vi "AO CorrLoop_PD_2D_v1.vi"() -> ()   [LabVIEW 2018]
uses:
  Casao LabVIEW SDK 1.0.5/Casao/Casao/Casao.ctl
  <vilib>/Analysis/1siggen.llb/Ramp Pattern by Samples.vi
  <vilib>/Utility/file.llb/Read From Spreadsheet File (DBL).vi
  <vilib>/Analysis/1siggen.llb/Ramp Pattern by Delta.vi
  <vilib>/Analysis/NI_AALBase.lvlib
panel:
  in  "Output Path 2":path=path "F:/Data_Min"
  in  "Trigger EMCCD":bool
  out "Tab Control":T1(tab)
  in  "Haso configuration file":path=path "C:/Program Files (x86)/Imagine Optic/Configuration Files/HASO3_first_7364.dat"
  in  "Offset command file":path=path "D:/SystemAlignment/system_aberration_20200627.dat"
  in  "Initial haso file":path=path "D:/SystemAlignment/system_aberration_residual_20200711.has"
  in  "EMCCD trigger port":tag="Dev1/port0/line0"
  out "Casao Index":T2
  out "# of Phase":i32
  in  "Error in":errorcluster
  in  "COMMAND matrix file":path=path "D:/SystemAlignment/CM_20200711_0p5x6.aomc"
  out "Error out":errorcluster
  in  "Diversity Zern Coeffs":enum16{"Manual ", "ZernFile"}(ring)=enum."ZernFile"
  in  "Zern coeffs initial":dbl[](array[numeric])=[0.3, 0.0]
  in  "Zern index initial":dbl[](array[numeric])=[4.0, 0.0]
  out "Zern coeffs (random)":dbl[](array[numeric])
  out "Zern index  (random from 4th)":dbl[](array[numeric])
  in  "aberration tolerance":dbl=0.1 format="%#_13g"
  in  "aberration threshold":dbl=0.25 format="%#_13g"
  in  "Initial Zern Coeffs":enum16{"Manual ", "Random"}(ring)
  in  "max random index":i64=9
  in  "Exp Repeat Num":i32=1
  in  "Coeffs 5":sgl[](array[numeric])=[-0.2, 0.5, 0.0, 0.0, 0.0, -0.2]
  in  "Index 5":i32[](array[numeric])=[3, 4, 5, 6, 7, 8]
  in  "Coeffs 4":sgl[](array[numeric])=[0.2, -0.5, 0.0, 0.0, 0.0, 0.0]
  in  "Index 4":i32[](array[numeric])=[3, 4, 5, 6, 7, 8]
  in  "Coeffs 3":sgl[](array[numeric])=[-0.2, -0.5, 0.0, 0.0, 0.0, 0.0]
  in  "Index 3":i32[](array[numeric])=[3, 4, 5, 6, 7, 8]
  in  "Coeffs 2":sgl[](array[numeric])=[0.2, 0.5, 0.0, 0.0, 0.0, 0.0]
  in  "Index 2":i32[](array[numeric])=[3, 4, 5, 6, 7, 8]
  in  "Zern coeffs file":path=path "D:/SystemAlignment/system_aberration_residual_20200711.txt"
  in  "Subfolder":string="Sample1"
  out "RMSE Value":dbl
  out "Time cost (s)":dbl
  in  "Folder Name":string="Test"
  in  "Main Path":path=path "D:/Data"
  in  "File Base Name":string="beads_test"
  in  "Images/phase":dbl=1.0
  in  "Exposure time (s)":string="0.02"
  in  "Num of Accumulations":string="1"
  in  "Diversity Phase Num":i32=2
  in  "ROI size":enum16{"full (1002*1002)", "512*512"}(ring)
  in  "take offset image?":bool=TRUE
  in  "Keep Reconstructed Defocus component?":bool caption="Apply Defocus"
  in  "PD Correction":bool=TRUE
  in  "Calculation Phase Num":u32=2
  in  "Number for average":u32=1
  in  "Zernike Index Limit":u32=21
  in  "Iteration Number":u32=10
  in  "Gamma Value":dbl=1e-06
  in  "Crop Size of image":u32=512
  in  "Background Value":u32=310
  in  "Show Input":bool
  in  "Show Recon":bool=TRUE
  in  "Use GPU":bool=TRUE
  # "AO correction loop based on phase diversity: 2D image case\nVersion 1: A combination of LabVIEW, MATLAB, and Andor software(by triggers)\n1) Replaced CASAO SDK function by new WaveTune SDK function;\n2) Reorgized UI and file/folder name;\n3) New PD recon MATLAB code (termination criterion)"
  # "How to use (date: 20200711)\n1) Run this VI;\n2) Run Andor script: AO CorrLoop_PD_2D_v1_Script\n3) Click \"Start Acquisition\" button."
  # "Manual input"
  # "Random input"
  # "Manual input sequence"
  # "File input"
  # "Path and File Name"
  # "Camera Preview"
  # "Andor EMCCD Settings"
  # "Module to add"
  # "Image Metrics"
  # "MATLAB Settings"
  # "Module to add"
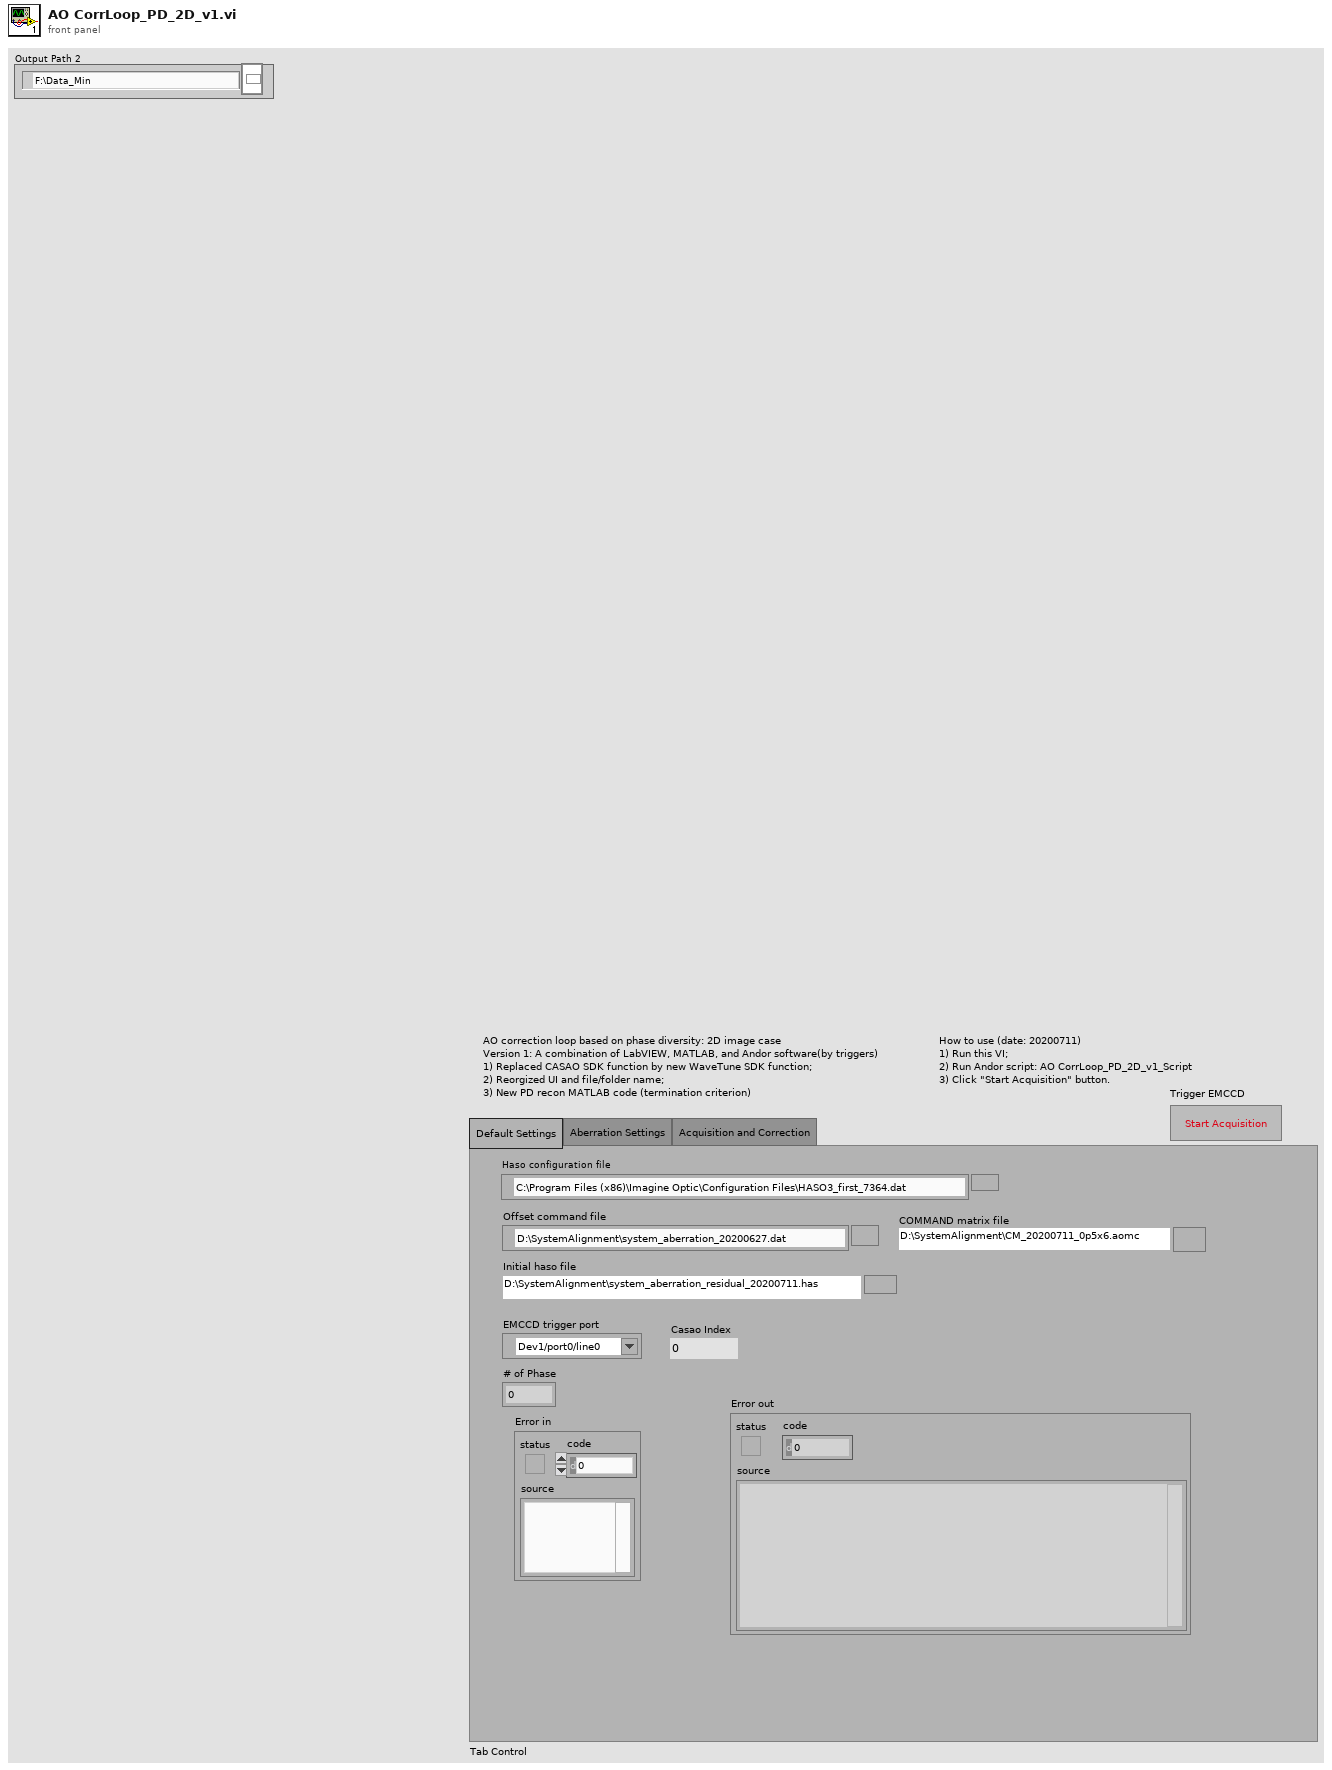
[diagram p1: front panel]
types:
  T1 = enum32{"Default Settings", "Aberration Settings", "Acquisition and Correction"}
  T2 = typedef "Casao.ctl" = i32
  T3 = typedef "PhaseModul.ctl" = i32
  T4 = typedef "NI_Matrix.lvlib/RealMatrix.ctl" = dbl[][]
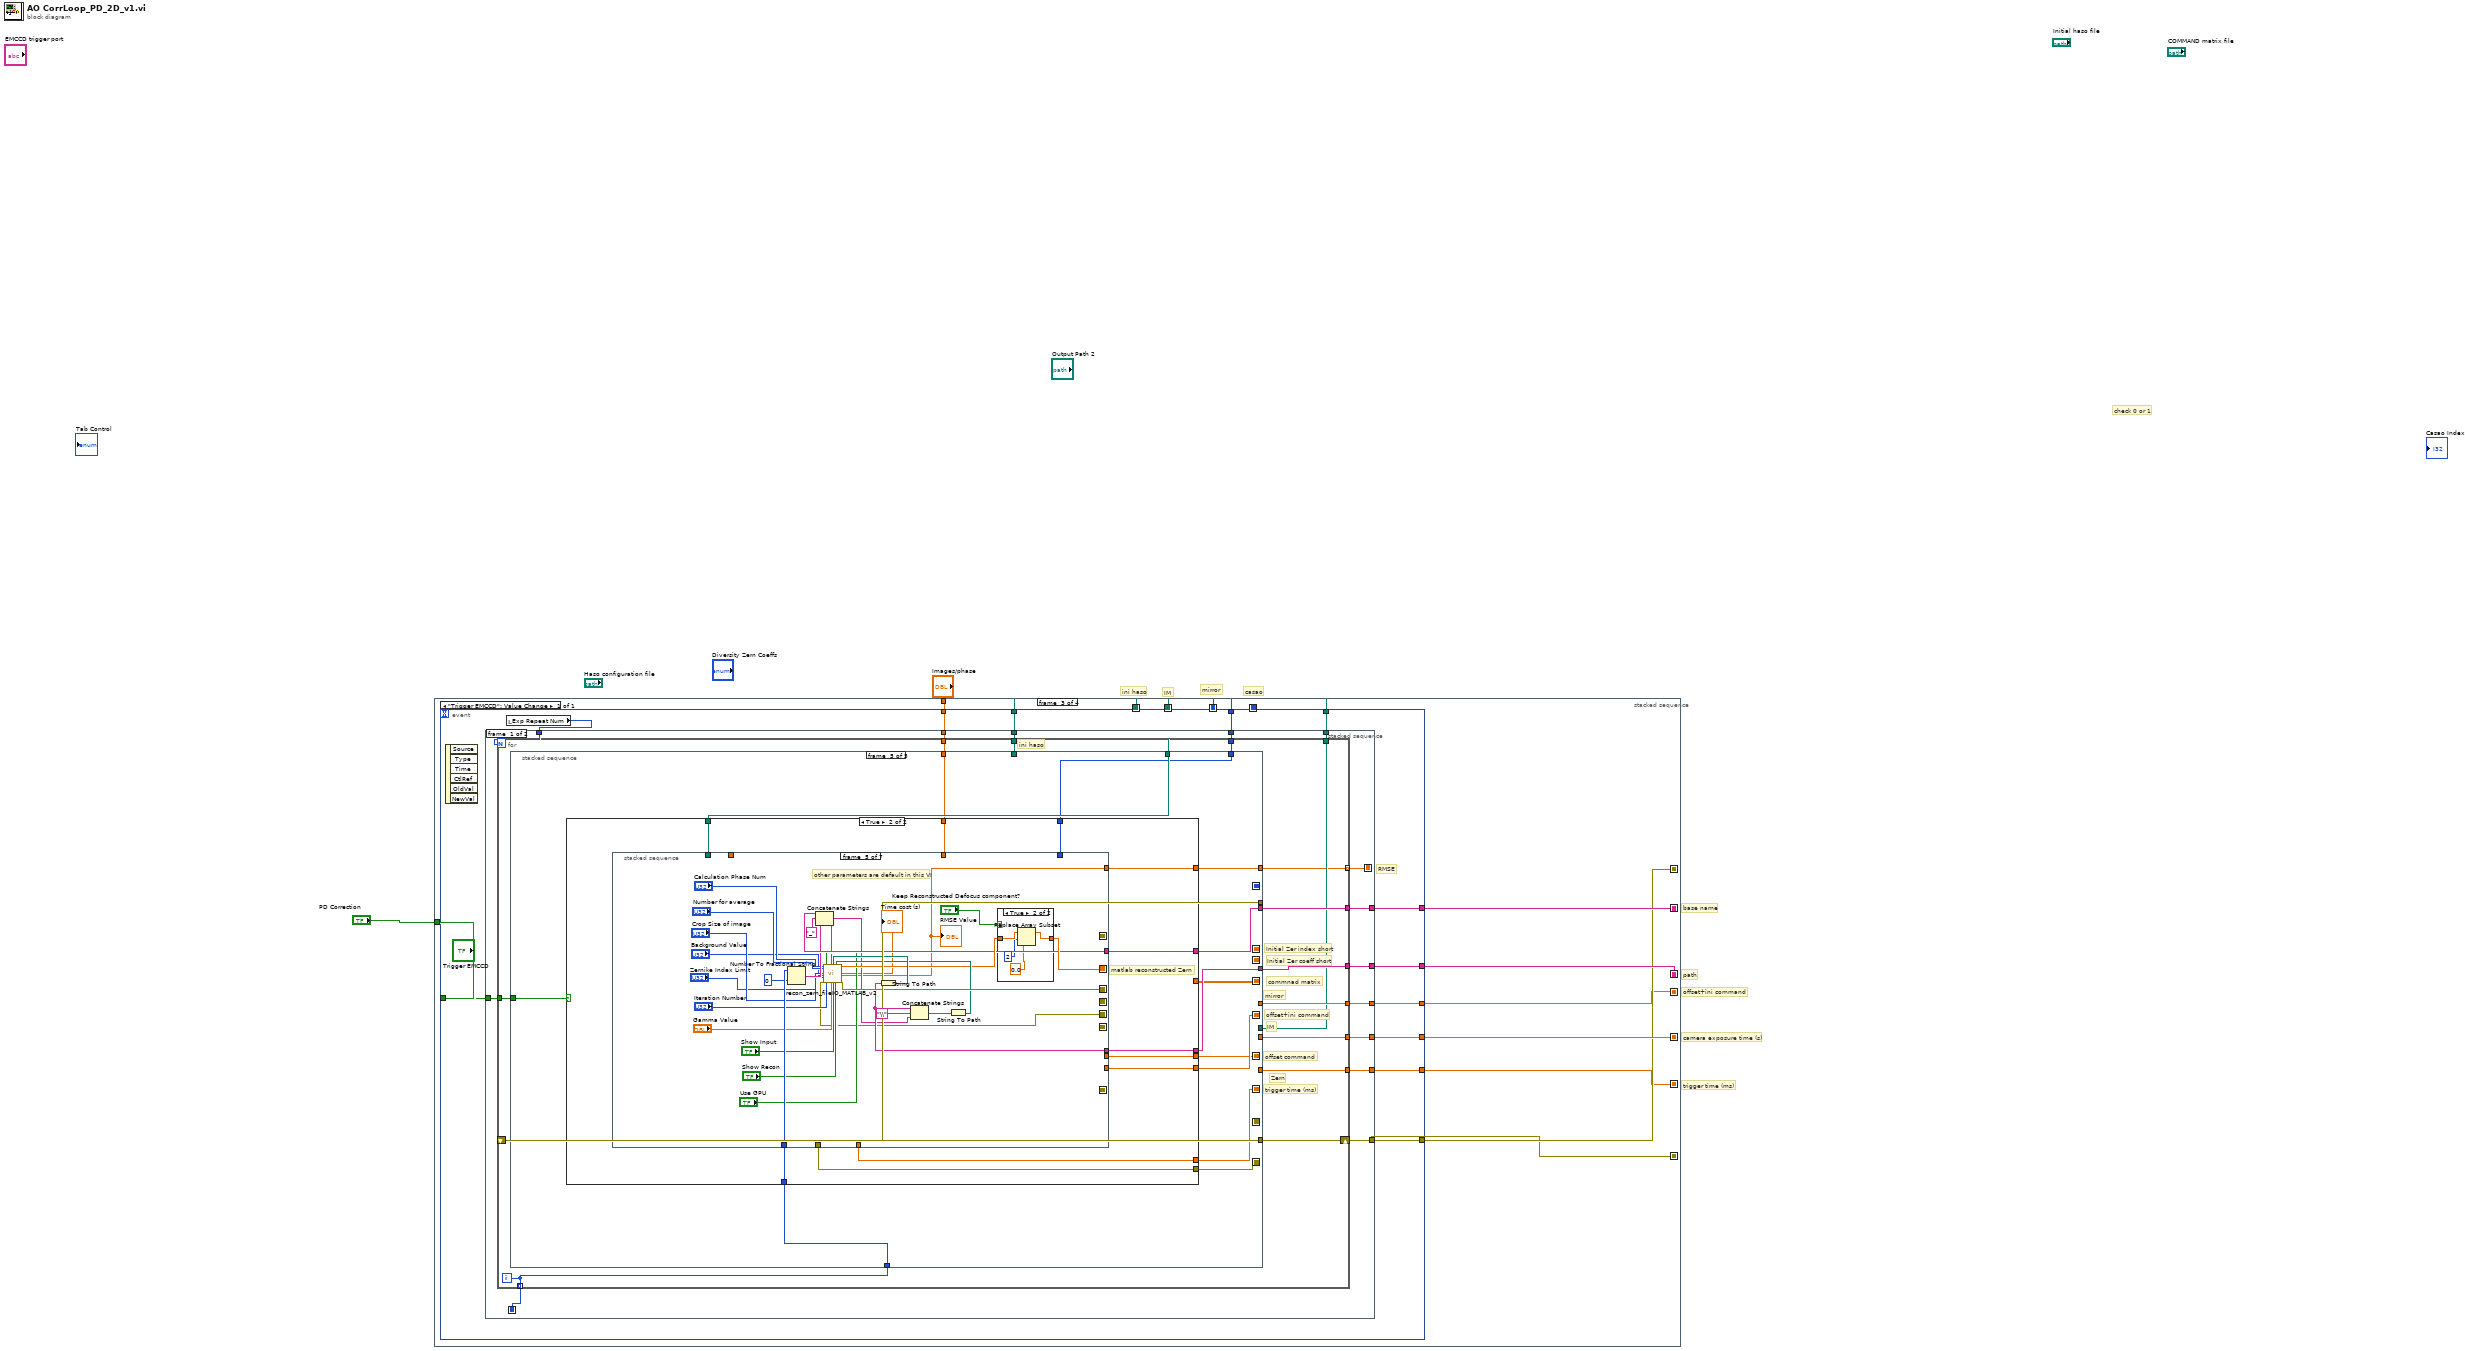
[diagram p0: block diagram]
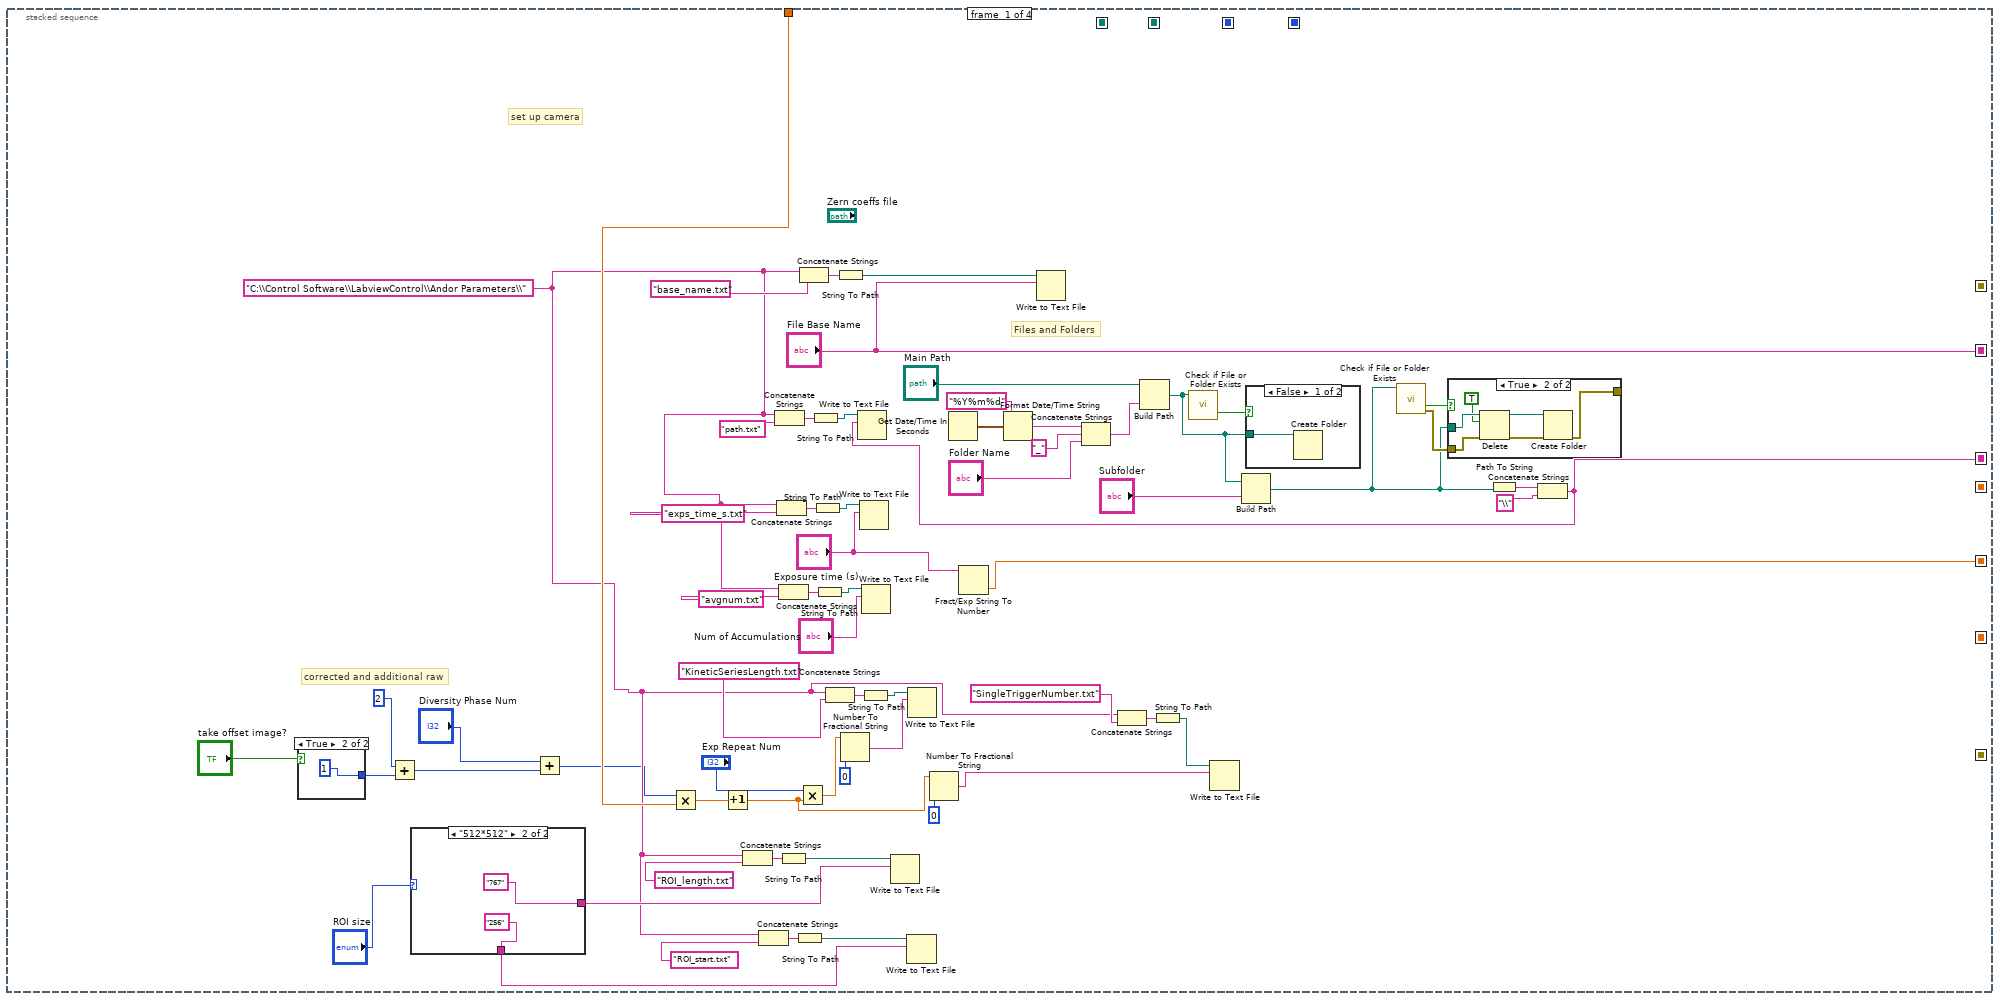
[diagram p2: hidden frame]
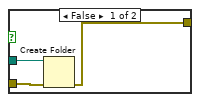
[diagram p3: hidden frame]
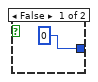
[diagram p5: hidden frame]
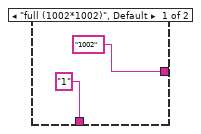
[diagram p6: hidden frame]
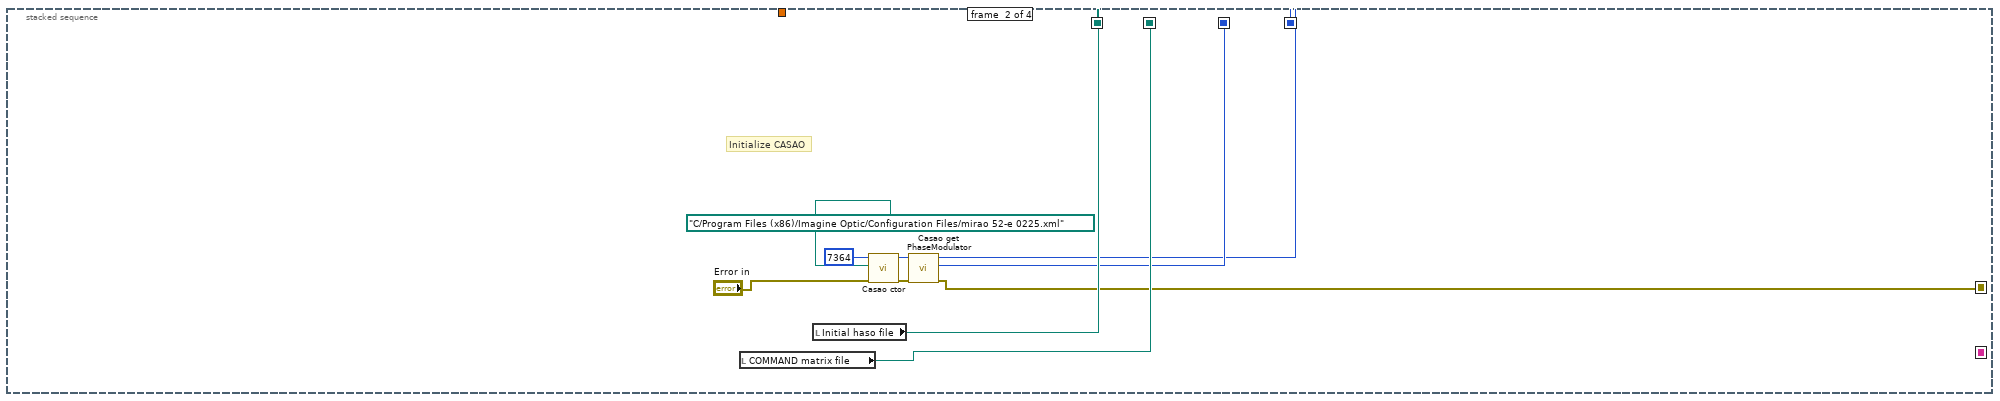
[diagram p7: hidden frame]
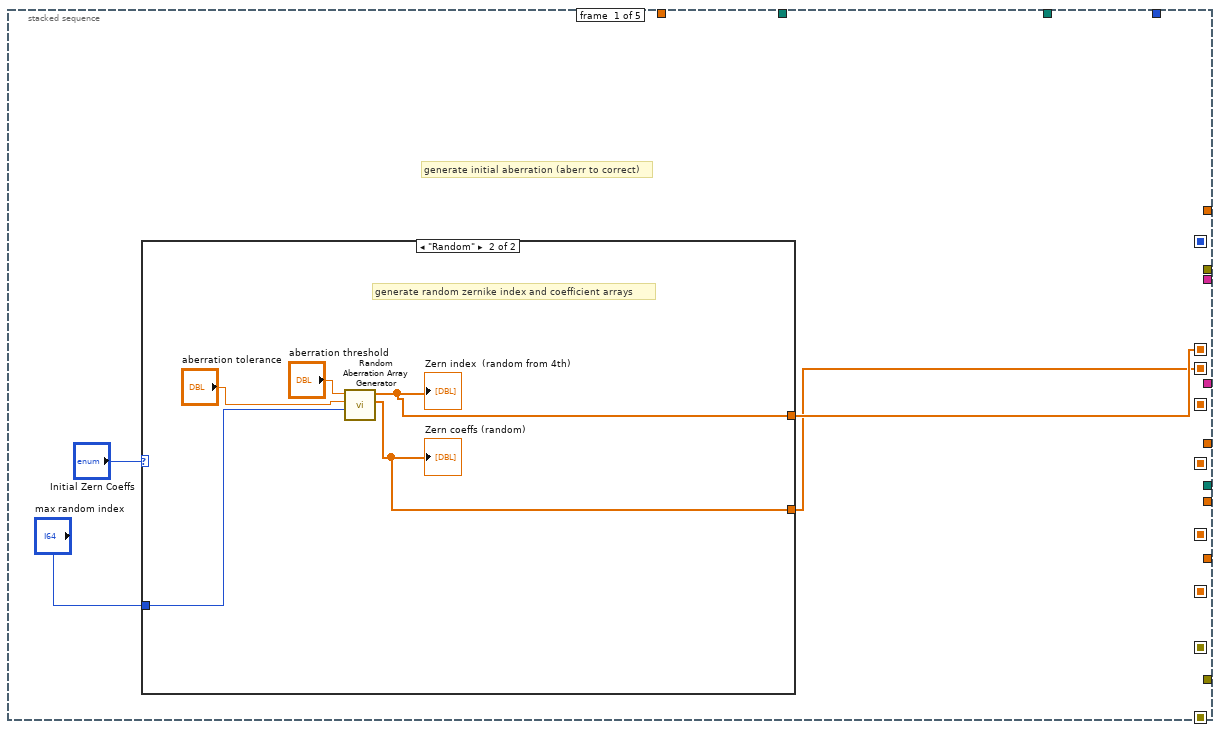
[diagram p8: hidden frame]
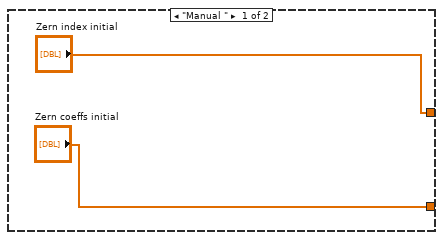
[diagram p9: hidden frame]
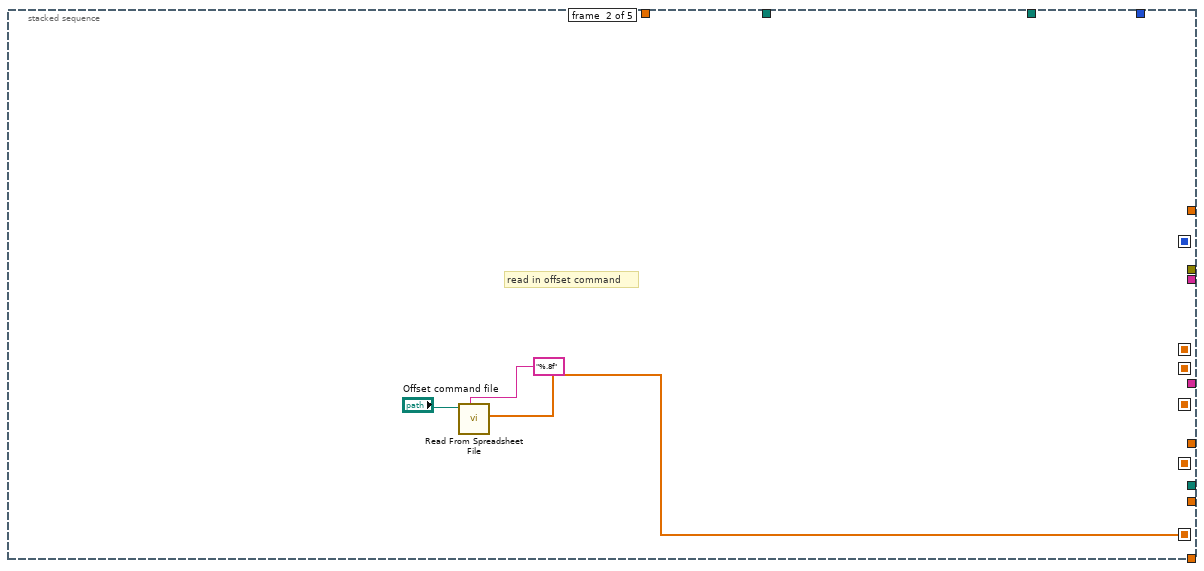
[diagram p10: hidden frame]
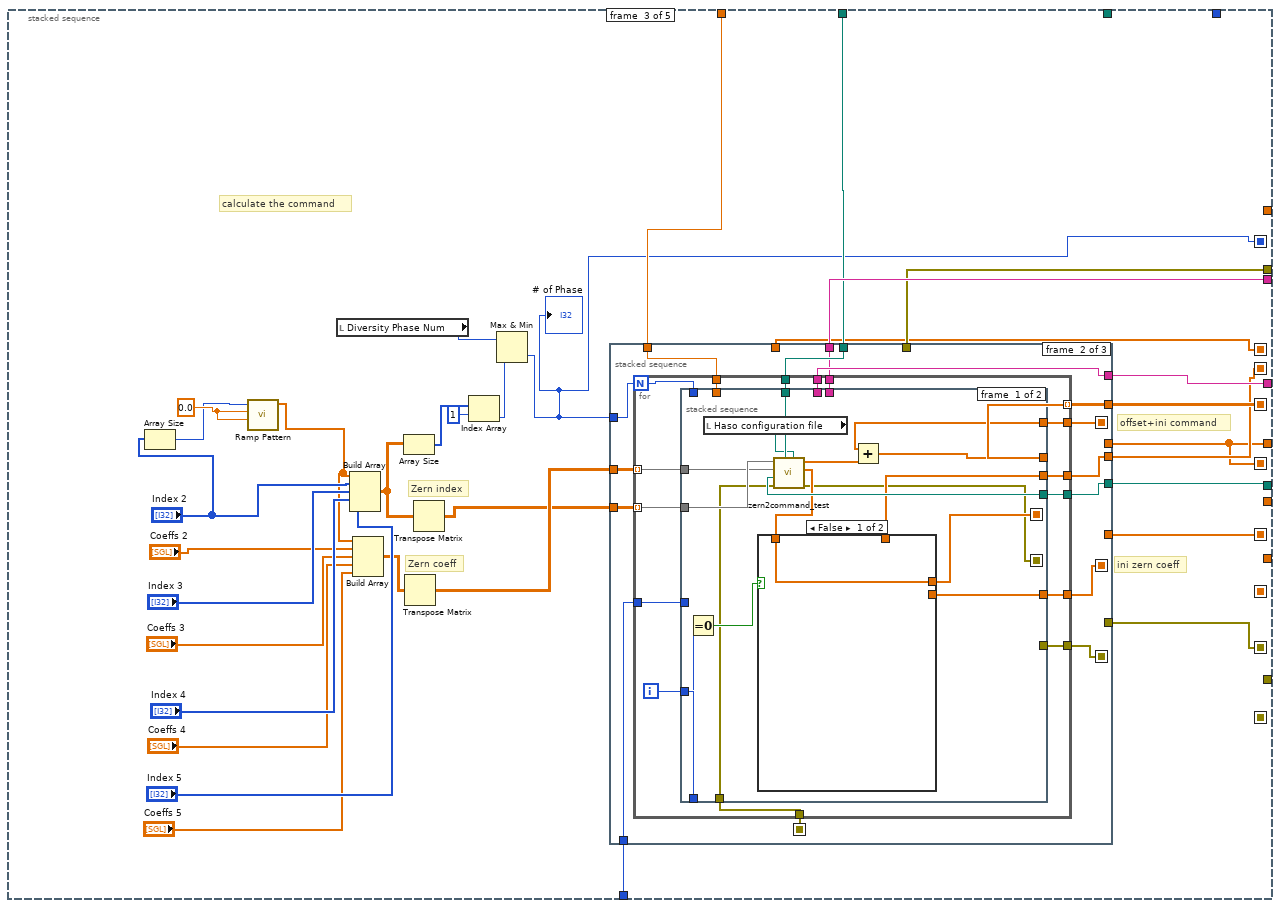
[diagram p11: hidden frame]
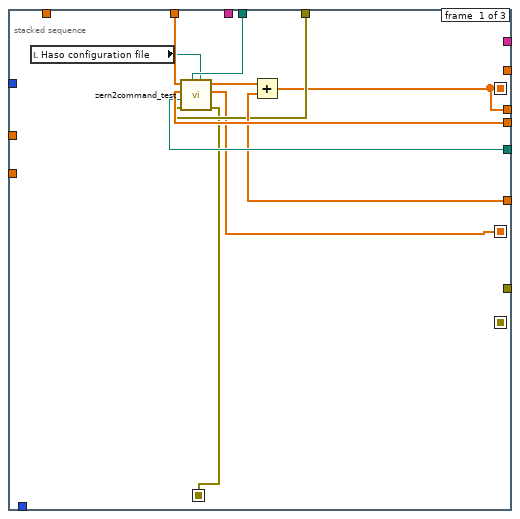
[diagram p12: hidden frame]
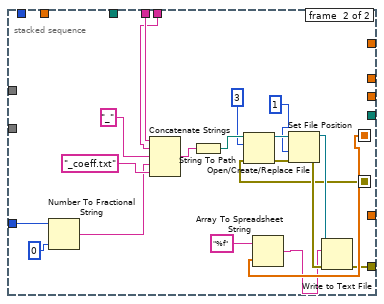
[diagram p14: hidden frame]
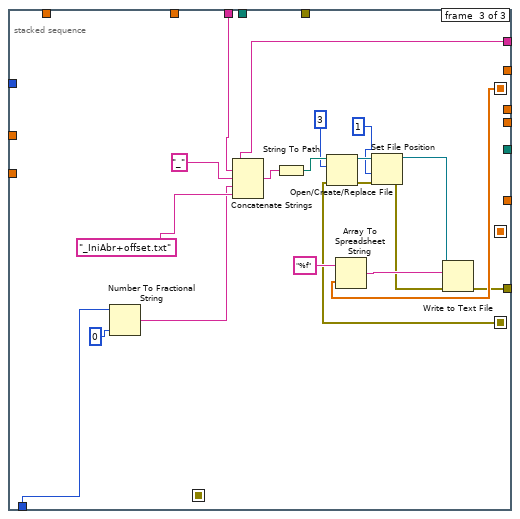
[diagram p15: hidden frame]
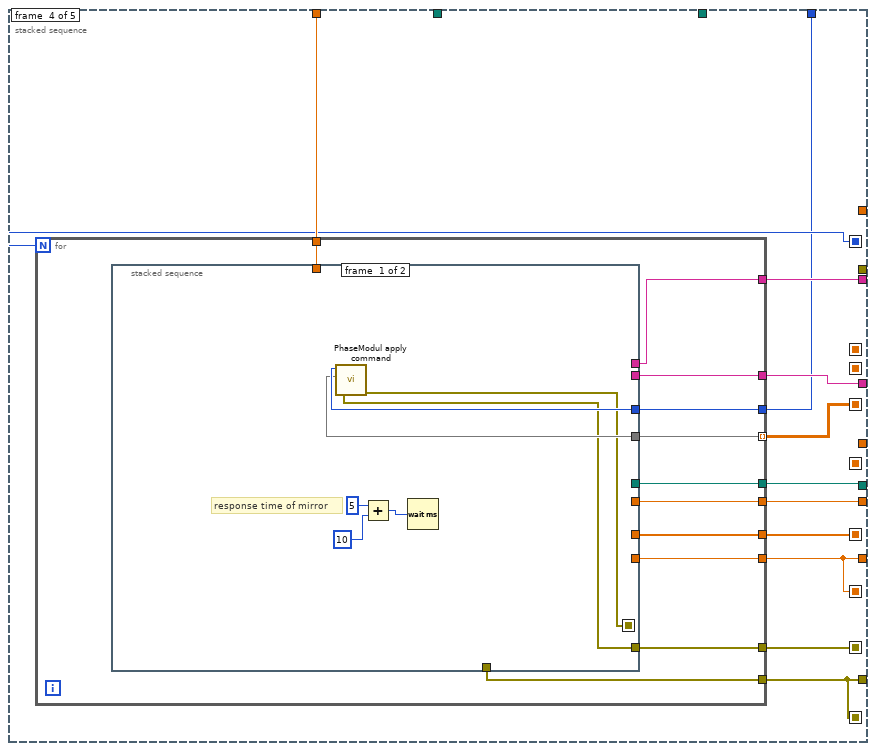
[diagram p16: hidden frame]
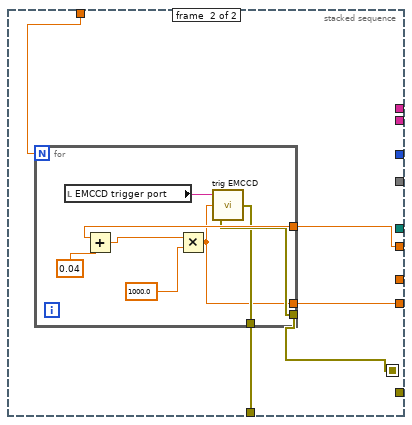
[diagram p17: hidden frame]
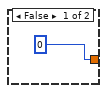
[diagram p18: hidden frame]
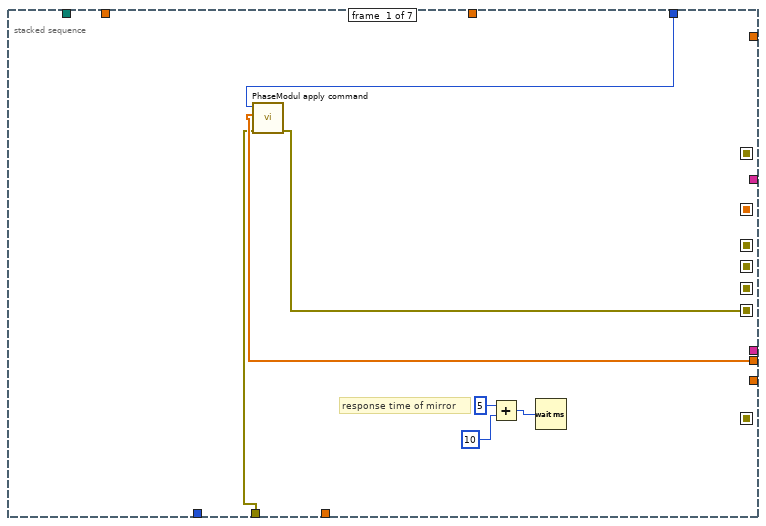
[diagram p19: hidden frame]
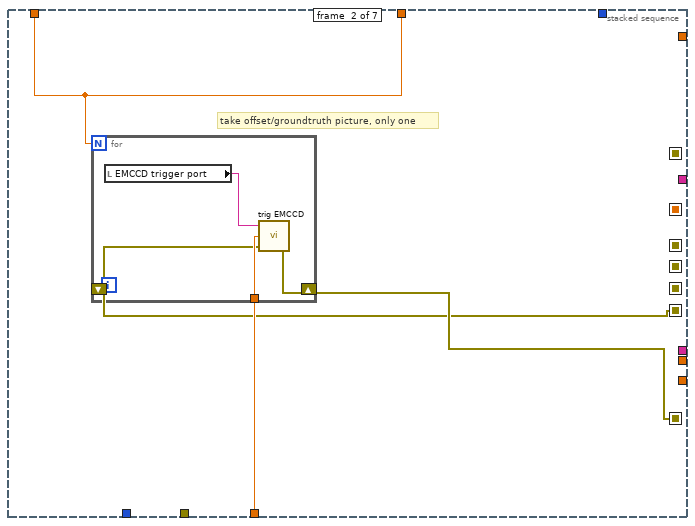
[diagram p20: hidden frame]
diagram:
  # "trigger time (ms)"
  # "offset+ini command"
  # "camera exposure time (s)"
  # "casao"
  # "mirror"
  # "IM"
  # "ini haso"
  # "path"
  # "base name"
  # "check 0 or 1"
  n1 = stacked-sequence {
    seq-local: [w3 _ _ _] -> [_ _ w102 _]
    seq-local: ["File Base Name" _ _ _] -> [_ _ w101 _]
    seq-local: [_ w87 _ _] -> [_ _ w99 _]
    seq-local: [_ w86 _ _] -> [_ _ w93 _]
    seq-local: [_ w85 _ _] -> [_ _ w100 _]
    seq-local: [_ w84 _ _] -> [_ _ _ w457]
    seq-local: [w37 _ _ _] -> [_ _ w98 _]
    seq-local: [_ w82 _ _] -> [_ _ w97 _]
    seq-local: [_ _ w96 _] -> [_ _ _ _]
    seq-local: [_ _ w95 _] -> [_ _ _ _]
    seq-local: [_ _ w94 _] -> [_ _ _ _]
    tunnel: "Images/phase" -> [w36 _ w103 _]
    tunnel: "PD Correction" -> [_ _ w92 _]
    frame #0 {
      w28 = "C:\\Control Software\\LabviewControl\\Andor Parameters\\"
      # "Files and Folders"
      # "corrected and additional raw"
      # "set up camera"
      n2 = case shown="True" "take offset image?" {
        tunnel: [0 1] -> w27
        frame False {
        }
        frame True {
        }
      }
      n3 = Add(x=2, y=w27) -> (x+y=w24:i32)
      n4 = case shown="\"512*512\"" "ROI size" {
        tunnel: ["1002" "767"] -> w43
        tunnel: ["1" "256"] -> w39
        frame "full (1002*1002)", Default {
        }
        frame "512*512" {
        }
      }
      n5 = Add(x="Diversity Phase Num", y=w24) -> (x+y=w22:i32)
      n6 = Multiply(x=w22, y=w36) -> (x*y=w20:dbl)
      n7 = Increment(x=w20) -> (x+1=w21:dbl)
      n8 = Concatenate Strings(w28, "ROI_length.txt") -> (w47:string)
      n9 = Concatenate Strings(w28, "ROI_start.txt") -> (w42:string)
      n10 = Concatenate Strings(w28, "path.txt") -> (w62:string)
      n11 = Concatenate Strings(w28, "exps_time_s.txt") -> (w59:string)
      n12 = Concatenate Strings(w28, "avgnum.txt") -> (w56:string)
      n13 = String To Path(string=w47) -> (path=w46:path)
      n14 = String To Path(string=w42) -> (path=w41:path)
      n15 = Multiply(x="Exp Repeat Num", y=w21) -> (x*y=w34:dbl)
      n16 = Concatenate Strings(w28, "base_name.txt") -> (w64:string)
      n17 = String To Path(string=w62) -> (path=w61:path)
      n18 = String To Path(string=w59) -> (path=w58:path)
      n19 = String To Path(string=w56) -> (path=w55:path)
      n20 = Concatenate Strings(w28, "KineticSeriesLength.txt") -> (w52:string)
      n21 = String To Path(string=w64) -> (path=w63:path)
      n22 = Number To Fractional String(number=w34, precision (6)=0) -> (F-format string=w49:string)  [unwired: 2 in]
      n23 = Write to Text File(file (use dialog)=w58, text="Exposure time (s)") -> ()  [unwired: 2 in, 3 out]
      n24 = Write to Text File(file (use dialog)=w55, text="Num of Accumulations") -> ()  [unwired: 2 in, 3 out]
      n25 = String To Path(string=w52) -> (path=w51:path)
      n26 = Write to Text File(file (use dialog)=w46, text=w43) -> ()  [unwired: 2 in, 3 out]
      n27 = Write to Text File(file (use dialog)=w41, text=w39) -> ()  [unwired: 2 in, 3 out]
      n28 = Write to Text File(file (use dialog)=w51, text=w49) -> ()  [unwired: 2 in, 3 out]
      n29 = Number To Fractional String(number=w21, precision (6)=0) -> (F-format string=w32:string)  [unwired: 2 in]
      n30 = Get Date/Time In Seconds() -> (seconds since 1Jan1904=w14:timestamp)
      n31 = Fract/Exp String To Number(string="Exposure time (s)") -> (number=w37:dbl)  [unwired: 3 in, 1 out]
      n32 = Format Date/Time String(time format string (%c)="%Y%m%d", seconds (now)=w14) -> (date/time string=w15:string)  [unwired: 1 in]
      n33 = Write to Text File(file (use dialog)=w63, text="File Base Name") -> ()  [unwired: 2 in, 3 out]
      n34 = Concatenate Strings(w15, "_", "Folder Name") -> (w16:string)
      n35 = Concatenate Strings(w28, "SingleTriggerNumber.txt") -> (w31:string)
      n36 = Build Path(base path="Main Path", name or relative path=w16) -> (appended path=w18:path)
      n37 = String To Path(string=w31) -> (path=w30:path)
      n38 = call <vilib>:"Check if File or Folder Exists.vi"("path"=w18) -> ("file or folder exists?"=w12:bool)  [unwired: 8 in, 2 out]
      n39 = Write to Text File(file (use dialog)=w30, text=w32) -> ()  [unwired: 2 in, 3 out]
      n40 = Build Path(base path=w18, name or relative path="Subfolder") -> (appended path=w4:path)
      n41 = case shown="False" w12 {
        tunnel: w18 -> [w75 _]
        frame False {
          n42 = Create Folder(path (use dialog)=w75) -> ()  [unwired: 2 in, 3 out]
        }
        frame True {
        }
      }
      n43 = call <vilib>:"Check if File or Folder Exists.vi"("path"=w4) -> ("error out"=w17:errorcluster, "file or folder exists?"=w13:bool)  [unwired: 8 in, 1 out]
      n44 = case shown="True" w13 {
        tunnel: w4 -> [w68 w73]
        tunnel: w17 -> [w67 w74]
        tunnel: [w66 w69] -> _
        frame False {
          n45 = Create Folder(path (use dialog)=w68, error in=w67) -> (error out=w66:errorcluster)  [unwired: 1 in, 2 out]
        }
        frame True {
          n46 = Delete(path (use dialog)=w73, entire hierarchy (F)=TRUE, error in=w74) -> (deleted path=w71:path, error out=w70:errorcluster)  [unwired: 2 in, 1 out]
          n47 = Create Folder(path (use dialog)=w71, error in=w70) -> (error out=w69:errorcluster)  [unwired: 1 in, 2 out]
        }
      }
      n48 = Path To String(path=w4) -> (string=w6:string)
      n49 = Concatenate Strings(w6, "\\") -> (w3:string)
      n50 = Write to Text File(file (use dialog)=w61, text=w3) -> ()  [unwired: 2 in, 3 out]
    }
    frame #1 {
      # "Initialize CASAO"
      n51 = local read "COMMAND matrix file"() -> (w86:path)
      n52 = local read "Initial haso file"() -> (w87:path)
      n53 = call "Casao ctor.vi"("error in (no error)"="Error in", "Mirror config file path"=path "C:/Program Files (x86)/Imagine Optic/Configuration Files/mirao 52-e 0225.xml", "Haso serial number"=u32 7364) -> ("error out"=w91:errorcluster, "Casao"=w90:T2)  [unwired: 5 in]
      n54 = call "Casao get PhaseModulator.vi"("error in (no error)"=w91, "Casao"=w90) -> ("error out"=w82:errorcluster, "Mirrror"=w85:T3, "Casao (dup)"=w84:T2)  [unwired: 3 in]
    }
    frame #2 {
      n55 = event shown="[0] \"Trigger EMCCD\": Value Change" {
        selector: _ -> [_]
        dyn-events: _ -> [_]
        timeout: _ -> [_]
        tunnel: w103 -> [w116]
        tunnel: w102 -> [w115]
        tunnel: w101 -> [w114]
        tunnel: w100 -> [w113]
        tunnel: w99 -> [w112]
        tunnel: w98 -> [w111]
        tunnel: w97 -> [w110]
        tunnel: [w109] -> w96
        tunnel: [w108] -> w95
        tunnel: [w107] -> w94
        tunnel: w93 -> [w106]
        tunnel: w92 -> [w105]
        event "Trigger EMCCD": Value Change {
          # "RMSE"
          n56 = event-data() -> ()  [unwired: 1 in, 6 out]
          n57 = local read "Exp Repeat Num"() -> (w104:i32)
          n58 = stacked-sequence {
            seq-local: [w118 _] -> [_ w452]
            seq-local: [w117 _] -> [_ _]
            tunnel: w116 -> [w131 _]
            tunnel: w115 -> [w130 w451]
            tunnel: w114 -> [w129 w450]
            tunnel: w113 -> [w128 _]
            tunnel: w112 -> [w127 _]
            tunnel: w111 -> [w126 _]
            tunnel: w110 -> [w125 _]
            tunnel: [w124 _] -> w109
            tunnel: [w123 _] -> w108
            tunnel: [w122 _] -> w107
            tunnel: w106 -> [w121 _]
            tunnel: w105 -> [w120 _]
            tunnel: w104 -> [w119 _]
            frame #0 {
              n59 = for {
                N: w119 -> [_]
                tunnel: w131 -> [w145]
                tunnel: w130 -> [w144]
                tunnel: w129 -> [w143]
                tunnel: w128 -> [w142]
                tunnel: w127 -> [w141]
                tunnel: w126 -> [w140]
                tunnel: [w138] -> w124
                tunnel: [w137] -> w123
                tunnel: w121 -> [w135]
                tunnel: w120 -> [w134]
                shift-right: [w136] -> w122
                shift-left: w125 -> [w139]
                tunnel: [w133] -> w118 mode=indexing
                tunnel: [w132] -> w117 mode=indexing
                i -> [w132]
                # "trigger time (ms)"
                # "offset+ini command"
                # "Initial Zer coeff short"
                # "Initial Zer index short"
                # "mirror"
                # "Zern"
                # "commnad matrix"
                # "ini haso"
                # "IM"
                # "offset command"
                n60 = stacked-sequence {
                  seq-local: [_ w157 _ _ _] -> [_ _ w179 w301 w336]
                  seq-local: [_ _ w177 _ _] -> [_ _ _ w300 w338]
                  seq-local: [_ _ w160 _ _] -> [_ _ _ w299 _]
                  seq-local: [_ _ w169 _ _] -> [_ _ _ w295 _]
                  seq-local: [w148 _ _ _ _] -> [_ _ w166 _ _]
                  seq-local: [w147 _ _ _ _] -> [_ _ w165 _ _]
                  seq-local: [_ _ w164 _ _] -> [_ _ _ _ w345]
                  seq-local: [_ _ _ w294 _] -> [_ _ _ _ w342]
                  seq-local: [_ _ _ w293 _] -> [_ _ _ _ w341]
                  tunnel: w145 -> [_ _ w173 w304 w343]
                  tunnel: w144 -> [_ _ w174 w303 w347]
                  tunnel: w143 -> [_ _ w175 w302 w348]
                  tunnel: w141 -> [_ _ w172 _ _]
                  tunnel: w135 -> [_ _ w171 w298 _]
                  tunnel: w142 -> [_ _ _ w297 w344]
                  tunnel: w140 -> [_ _ _ w296 _]
                  tunnel: w139 -> [_ _ w170 _ _]
                  tunnel: [_ _ _ w293 _] -> w136
                  tunnel: [_ _ w164 _ _] -> w138
                  tunnel: [_ _ _ w294 _] -> w137
                  tunnel: w135 -> [_ _ _ _ w346]
                  tunnel: w134 -> [_ _ _ _ w340]
                  tunnel: w132 -> [_ _ w163 _ w339]
                  tunnel: [_ _ _ _ w337] -> w133
                  frame #0 {
                    # "generate initial aberration (aberr to correct)"
                    n61 = case shown="\"Random\"" "Initial Zern Coeffs" {
                      tunnel: ["Zern index initial" w154] -> w148
                      tunnel: ["Zern coeffs initial" w153] -> w147
                      tunnel: "max random index" -> [_ w152]
                      frame "Manual " {
                      }
                      frame "Random" {
                        # "generate random zernike index and coefficient arrays"
                        n62 = call "Random Aberration Array Generator.vi"("max random order"=w152, "aberration tolerance"="aberration tolerance", "aberration threshold"="aberration threshold") -> ("Zer coeff"=w153:dbl[], "Zer index (starting from 3)"=w154:dbl[])  [unwired: 7 in]
                        "Zern index  (random from 4th)" <- w154
                        "Zern coeffs (random)" <- w153
                      }
                    }
                  }
                  frame #1 {
                    # "read in offset command"
                    n63 = call-poly <vilib>:"Read From Spreadsheet File.vi"("format (%.3f)"="%.8f", "file path (dialog if empty)"="Offset command file") -> ("first row"=w157:dbl[])  [unwired: 5 in, 4 out]
                  }
                  frame #2 {
                    w184 = 0.0
                    # "ini zern coeff"
                    # "offset+ini command"
                    # "Zern coeff"
                    # "Zern index"
                    # "calculate the command"
                    n64 = Array Size(array="Index 2") -> (size(s)=w182:i32)
                    n65 = call-poly <vilib>:"Ramp Pattern.vi"("start"=w184, "end"=w184, "samples"=w182) -> ("Ramp Pattern"=w181:dbl[])  [unwired: 7 in, 1 out]
                    n66 = local read "Diversity Phase Num"() -> (w162:i32)
                    n67 = Build Array(w181, "Index 2", "Index 3", "Index 4", "Index 5") -> (w167:T4)
                    n68 = Build Array(w181, "Coeffs 2", "Coeffs 3", "Coeffs 4", "Coeffs 5") -> (w185:T4)
                    n69 = Array Size(array=w167) -> (size(s)=w168:i32[])
                    n70 = Transpose Matrix(1:w185) -> (0:w178:T4)
                    n71 = Transpose Matrix(1:w167) -> (0:w176:T4)
                    n72 = Index Array(array=w168, index=1) -> (element=w161:i32)
                    n73 = Max & Min(x=w162, y=w161) -> (min(x,y)=w160:i32)  [unwired: 1 out]
                    "# of Phase" <- w160
                    n74 = stacked-sequence {
                      seq-local: [w195 _ _] -> [_ w213 w280]
                      seq-local: [w196 _ _] -> [_ w207 _]
                      seq-local: [_ w206 _] -> [_ _ w277]
                      seq-local: [w194 _ _] -> [_ w205 _]
                      tunnel: w160 -> [_ w218 _]
                      tunnel: w166 -> [w203 _ _]
                      tunnel: w165 -> [w202 w208 _]
                      tunnel: w171 -> [w201 w215 _]
                      tunnel: w179 -> [w199 _ _]
                      tunnel: w176 -> [_ w217 _]
                      tunnel: w178 -> [_ w216 _]
                      tunnel: w172 -> [w198 w214 _]
                      tunnel: [_ w212 _] -> w177
                      tunnel: w175 -> [_ w210 w278]
                      tunnel: w174 -> [_ w211 w279]
                      tunnel: w173 -> [_ w209 _]
                      tunnel: w170 -> [w197 _ _]
                      tunnel: [_ _ w276] -> w169
                      tunnel: [w195 _ _] -> w164
                      tunnel: w163 -> [_ w204 w274]
                      frame #0 {
                        n75 = local read "Haso configuration file"() -> (w193:path)
                        n76 = call "zern2command_test.vi"("Haso configuration file"=w193, "Initial haso file"=w198, "error in (no error)"=w197, "interaction matrix file"=w201, "Zern coef in"=w202, "Zern index in"=w203) -> ("error out"=w196:errorcluster, "Zern coef out"=w194:sgl[], "Offset positions"=w200:sgl[])  [unwired: 3 in]
                        n77 = Add(x=w200, y=w199) -> (x+y=w195:dbl[])
                      }
                      frame #1 {
                        n78 = for {
                          N: w218 -> [w221]
                          tunnel: w217 -> [w234] mode=indexing
                          tunnel: w216 -> [w233] mode=indexing
                          tunnel: w215 -> [w232]
                          tunnel: w214 -> [w231]
                          tunnel: w213 -> [w230]
                          tunnel: [w229] -> w212 mode=indexing
                          tunnel: w211 -> [w228]
                          tunnel: w210 -> [w227]
                          tunnel: w209 -> [w226]
                          tunnel: w208 -> [w225]
                          tunnel: w207 -> [w224]
                          tunnel: [w223] -> w206
                          tunnel: w205 -> [w220]
                          tunnel: w204 -> [w219]
                          i -> [w222]
                          n79 = stacked-sequence {
                            seq-local: [w241 _] -> [_ w260]
                            seq-local: [w237 _] -> [_ w259]
                            tunnel: w234 -> [w250 _]
                            tunnel: w233 -> [w249 _]
                            tunnel: w232 -> [w248 _]
                            tunnel: w231 -> [w247 _]
                            tunnel: w230 -> [w245 _]
                            tunnel: [w244 _] -> w229
                            tunnel: w228 -> [_ w262]
                            tunnel: w227 -> [_ w261]
                            tunnel: w226 -> [_ _]
                            tunnel: w222 -> [w243 _]
                            tunnel: w225 -> [w239 _]
                            tunnel: w224 -> [w238 _]
                            tunnel: [_ w258] -> w223
                            tunnel: w222 -> [_ _]
                            tunnel: w221 -> [_ _]
                            tunnel: w220 -> [w236 _]
                            tunnel: w219 -> [_ w255]
                            frame #0 {
                              n80 = Equal To 0?(x=w243) -> (x = 0?=w242:bool)
                              n81 = local read "Haso configuration file"() -> (w235:path)
                              n82 = call "zern2command_test.vi"("Haso configuration file"=w235, "Initial haso file"=w247, "error in (no error)"=w238, "interaction matrix file"=w248, "Zern coef in"=w249, "Zern index in"=w250) -> ("error out"=w237:errorcluster, "Zern coef out"=w240:sgl[], "Offset positions"=w246:sgl[])  [unwired: 3 in]
                              n83 = case shown="False" w242 {
                                tunnel: [w251 w252] -> w241
                                tunnel: w240 -> [w251 _]
                                tunnel: w239 -> [_ _]
                                tunnel: w236 -> [_ w252]
                                frame False {
                                }
                                frame True {
                                }
                              }
                              n84 = Add(x=w245, y=w246) -> (x+y=w244:dbl[])
                            }
                            frame #1 {
                              n85 = Number To Fractional String(number=w255, precision (6)=0) -> (F-format string=w254:string)  [unwired: 2 in]
                              n86 = Concatenate Strings(w262, w261, "_", w254, "_coeff.txt") -> (w270:string)
                              n87 = String To Path(string=w270) -> (path=w269:path)
                              n88 = Open/Create/Replace File(file path (use dialog)=w269, error in=w259, operation (0:open)=3) -> (refnum out=w266:refnum<file>, error out=w267:errorcluster)  [unwired: 3 in, 1 out]
                              n89 = Array To Spreadsheet String(array=w260, 3:"%f") -> (spreadsheet string=w257:string)  [unwired: 1 in]
                              n90 = Set File Position(refnum=w266, from (0:start)=1, error in=w267) -> (refnum out=w264:refnum<file>, error out=w263:errorcluster)  [unwired: 1 in]
                              n91 = Write to Text File(file (use dialog)=w264, text=w257, error in=w263) -> (error out=w258:errorcluster)  [unwired: 1 in, 2 out]
                            }
                          }
                        }
                      }
                      frame #2 {
                        n92 = Number To Fractional String(number=w274, precision (6)=0) -> (F-format string=w273:string)  [unwired: 2 in]
                        n93 = Concatenate Strings(w279, w278, "_", w273, "_IniAbr+offset.txt") -> (w289:string)
                        n94 = String To Path(string=w289) -> (path=w287:path)
                        n95 = Open/Create/Replace File(file path (use dialog)=w287, error in=w277, operation (0:open)=3) -> (refnum out=w284:refnum<file>, error out=w285:errorcluster)  [unwired: 3 in, 1 out]
                        n96 = Array To Spreadsheet String(array=w280, 3:"%f") -> (spreadsheet string=w291:string)  [unwired: 1 in]
                        n97 = Set File Position(refnum=w284, from (0:start)=1, error in=w285) -> (refnum out=w282:refnum<file>, error out=w281:errorcluster)  [unwired: 1 in]
                        n98 = Write to Text File(file (use dialog)=w282, text=w291, error in=w281) -> (error out=w276:errorcluster)  [unwired: 1 in, 2 out]
                      }
                    }
                  }
                  frame #3 {
                    n99 = for {
                      N: w299 -> [_]
                      tunnel: w304 -> [w315]
                      tunnel: w303 -> [w314]
                      tunnel: w302 -> [w313]
                      tunnel: w298 -> [w312]
                      tunnel: w301 -> [w311]
                      tunnel: w297 -> [w310]
                      tunnel: w300 -> [w309] mode=indexing
                      tunnel: w296 -> [w308]
                      tunnel: w295 -> [w307]
                      tunnel: [w306] -> w293
                      tunnel: [w305] -> w294
                      n100 = stacked-sequence {
                        seq-local: [w316 _] -> [_ w325]
                        tunnel: w315 -> [_ w327]
                        tunnel: w314 -> [_ _]
                        tunnel: w313 -> [_ _]
                        tunnel: w312 -> [_ _]
                        tunnel: w311 -> [_ _]
                        tunnel: w310 -> [w322 _]
                        tunnel: w309 -> [w321 _]
                        tunnel: w308 -> [_ w326]
                        tunnel: w307 -> [w317 _]
                        tunnel: [_ w324] -> w306
                        tunnel: [_ w323] -> w305
                        frame #0 {
                          # "response time of mirror"
                          n101 = call "PhaseModul apply command.vi"("error in (no error)"=w317, "Commands in"=w321, "Mirror"=w322) -> ("error out"=w316:errorcluster)  [unwired: 2 in, 2 out]
                          n102 = Add(x=5, y=10) -> (x+y=w318:i32)
                          n103 = Wait (ms)(milliseconds to wait=w318) -> ()  [unwired: 1 out]
                        }
                        frame #1 {
                          n104 = for {
                            N: w327 -> [_]
                            tunnel: w326 -> [w332]
                            tunnel: w325 -> [w330]
                            tunnel: [w329] -> w324
                            tunnel: [w328] -> w323
                            n105 = local read "EMCCD trigger port"() -> (w335:tag)
                            n106 = Add(x=w332, y=0.04) -> (x+y=w331:dbl)
                            n107 = Multiply(x=w331, y=1000.0) -> (x*y=w328:dbl)
                            n108 = call "trig EMCCD.vi"("error in (no error)"=w330, "exp time (ms)"=w328, "lines"=w335) -> ("error out"=w329:errorcluster)
                          }
                        }
                      }
                    }
                  }
                  frame #4 {
                    n109 = case shown="True" w340 {
                      tunnel: w347 -> [_ w360]
                      tunnel: w348 -> [_ w359]
                      tunnel: w346 -> [_ w358]
                      tunnel: w345 -> [_ w357]
                      tunnel: w344 -> [_ w356]
                      tunnel: w342 -> [_ w355]
                      tunnel: w343 -> [_ w354]
                      tunnel: w341 -> [_ w353]
                      tunnel: w339 -> [_ w352]
                      tunnel: w338 -> [_ _]
                      tunnel: [0 w351] -> w337
                      tunnel: w336 -> [_ w350]
                      frame False {
                      }
                      frame True {
                        # "matlab reconstructed Zern"
                        n110 = stacked-sequence {
                          seq-local: [_ _ _ _ w410 _ _] -> [_ _ _ _ _ w437 _]
                          seq-local: [_ _ _ _ w417 _ _] -> [_ _ _ _ _ w428 _]
                          seq-local: [_ _ w376 _ _ _ _] -> [_ _ _ w385 _ _ _]
                          seq-local: [w366 _ _ _ _ _ _] -> [_ w369 _ _ _ _ _]
                          seq-local: [_ w370 _ _ _ _ _] -> [_ _ w380 _ _ _ _]
                          seq-local: [_ _ _ w384 _ _ _] -> [_ _ _ _ w394 _ _]
                          seq-local: [_ _ _ _ _ w430 _] -> [_ _ _ _ _ _ w443]
                          tunnel: w360 -> [_ _ _ _ w416 _ _]
                          tunnel: w359 -> [_ _ _ _ w409 _ _]
                          tunnel: w358 -> [_ _ _ _ _ w436 _]
                          tunnel: w357 -> [_ _ w381 _ _ w429 _]
                          tunnel: w356 -> [w367 _ w382 _ _ w435 _]
                          tunnel: w355 -> [_ w371 _ w386 _ _ w445]
                          tunnel: w353 -> [w361 _ _ _ _ _ _]
                          tunnel: [_ w368 _ _ _ _ _] -> _
                          tunnel: w354 -> [_ w368 _ w383 _ _ w441]
                          tunnel: w352 -> [_ _ _ _ w408 _ _]
                          tunnel: [_ _ _ _ w391 _ _] -> w351
                          tunnel: w350 -> [w365 _ _ _ _ _ _]
                          frame #0 {
                            # "response time of mirror"
                            n111 = call "PhaseModul apply command.vi"("error in (no error)"=w361, "Commands in"=w365, "Mirror"=w367) -> ("error out"=w366:errorcluster)  [unwired: 2 in, 2 out]
                            n112 = Add(x=5, y=10) -> (x+y=w362:i32)
                            n113 = Wait (ms)(milliseconds to wait=w362) -> ()  [unwired: 1 out]
                          }
                          frame #1 {
                            # "take offset/groundtruth picture, only one"
                            n114 = for {
                              N: w368 -> [_]
                              tunnel: w371 -> [w375]
                              shift-right: [w374] -> w370
                              shift-left: w369 -> [w372]
                              n115 = local read "EMCCD trigger port"() -> (w373:tag)
                              n116 = call "trig EMCCD.vi"("error in (no error)"=w372, "exp time (ms)"=w375, "lines"=w373) -> ("error out"=w374:errorcluster)
                            }
                          }
                          frame #2 {
                            # "response time of mirror"
                            n117 = call "PhaseModul apply command.vi"("error in (no error)"=w380, "Commands in"=w381, "Mirror"=w382) -> ("error out"=w376:errorcluster)  [unwired: 2 in, 2 out]
                            n118 = Add(x=5, y=10) -> (x+y=w377:i32)
                            n119 = Wait (ms)(milliseconds to wait=w377) -> ()  [unwired: 1 out]
                          }
                          frame #3 {
                            # "take offset+initial aberr picture, only one"
                            n120 = for {
                              N: w383 -> [_]
                              tunnel: w386 -> [w390]
                              shift-right: [w387] -> w384
                              shift-left: w385 -> [w388]
                              n121 = local read "EMCCD trigger port"() -> (w389:tag)
                              n122 = call "trig EMCCD.vi"("error in (no error)"=w388, "exp time (ms)"=w390, "lines"=w389) -> ("error out"=w387:errorcluster)
                            }
                          }
                          frame #4 {
                            # "other parameters are default in this VI"
                            n123 = Number To Fractional String(number=w408, precision (6)=0) -> (F-format string=w406:string)  [unwired: 2 in]
                            n124 = Concatenate Strings(w409, "_", w406) -> (w395:string)
                            n125 = String To Path(string=w416) -> (path=w418:path)
                            n126 = Concatenate Strings(w416, "\\", w395) -> (w414:string)
                            n127 = String To Path(string=w414) -> (path=w413:path)
                            n128 = call "recon_zern_fileIO_MATLAB_v2.vi"("Number of Phase"="Calculation Phase Num", "Number for average"="Number for average", "Crop Size of image"="Crop Size of image", "Background Value"="Background Value", "Zernike Order"="Zernike Index Limit", "error in (no error)"=w394, "Use GPU"="Use GPU", "Iteration Number"="Iteration Number", "File Name"=w395, "Gamma Value"="Gamma Value", "Path In"=w418, "Show Input"="Show Input", "Path Out"=w413, "Show Recon"="Show Recon") -> ("Zern coef out"=w411:sgl[], "Time cost (s)"=→"Time cost (s)":dbl, "RMSE Value"=w391:dbl, "error out"=w417:errorcluster)  [unwired: 10 in]
                            "RMSE Value" <- w391
                            n129 = case shown="True" "Keep Reconstructed Defocus component?" {
                              tunnel: w411 -> [w419 w423]
                              tunnel: [w419 w420] -> w410
                              frame False {
                              }
                              frame True {
                                n130 = Replace Array Subset(array=w423, new element=0.0, index=2) -> (w420:sgl[])
                              }
                            }
                          }
                          frame #5 {
                            w440 = 1
                            # "response time of mirror"
                            n131 = local read "Initial haso file"() -> (w425:path)
                            n132 = call-poly <vilib>:"Ramp Pattern.vi"("start"=w440, "end"=32, "delta"=w440) -> ("Ramp Pattern"=w438:dbl[])  [unwired: 6 in, 2 out]
                            n133 = local read "Haso configuration file"() -> (w424:path)
                            n134 = call "zern2command_test.vi"("Haso configuration file"=w424, "Initial haso file"=w425, "error in (no error)"=w428, "interaction matrix file"=w436, "Zern coef in"=w437, "Zern index in"=w438) -> ("error out"=w426:errorcluster, "Offset positions"=w427:sgl[])  [unwired: 3 in, 1 out]
                            n135 = Add(x=w427, y=w429) -> (x+y=w434:dbl[])
                            n136 = call "PhaseModul apply command.vi"("error in (no error)"=w426, "Commands in"=w434, "Mirror"=w435) -> ("error out"=w430:errorcluster)  [unwired: 2 in, 2 out]
                            n137 = Add(x=5, y=10) -> (x+y=w431:i32)
                            n138 = Wait (ms)(milliseconds to wait=w431) -> ()  [unwired: 1 out]
                          }
                          frame #6 {
                            n139 = Increment(x=w441) -> (x+1=w442:dbl)
                            n140 = for {
                              N: w442 -> [_]
                              tunnel: w445 -> [w448]
                              shift-right: [w446] -> w444
                              shift-left: w443 -> [w447]
                              n141 = local read "EMCCD trigger port"() -> (w449:tag)
                              n142 = call "trig EMCCD.vi"("error in (no error)"=w447, "exp time (ms)"=w448, "lines"=w449) -> ("error out"=w446:errorcluster)
                            }
                            "Error out" <- w444
                          }
                        }
                      }
                    }
                  }
                }
              }
            }
            frame #1 {
              n143 = Concatenate Strings(w451, w450, "_RMSE.txt") -> (w456:string)
              n144 = String To Path(string=w456) -> (path=w455:path)
              n145 = Number To Fractional String(number=w452) -> (F-format string=w453:string[])  [unwired: 3 in]
              n146 = Write to Text File(file (use dialog)=w455, text=w453) -> ()  [unwired: 2 in, 3 out]
            }
          }
        }
      }
    }
    frame #3 {
      n147 = call "Casao dtor.vi"("Casao"=w457) -> ()  [unwired: 6 in, 1 out]
    }
  }
